vi "transparent IMAQ.vi"() -> ()   [LabVIEW 2015]
uses:
  <vilib>/vision/NI_Vision_Development_Module.lvlib
panel:
  in  "stop":bool
  in  "Transparency":dbl(slide) scale=0.0..100.0
  in  "Background":path=path "C:/Users/Public/Pictures/Sample Pictures/Chrysanthemum.jpg"
  in  "Overlay":path=path "C:/Users/ukrossk/Desktop/QuestionMark.png"
  out "Main Image":T1(plugin-control)
  out "Over Lay":T1(plugin-control)
  out "Image Out":T1(plugin-control)
  # "="
  # "+"
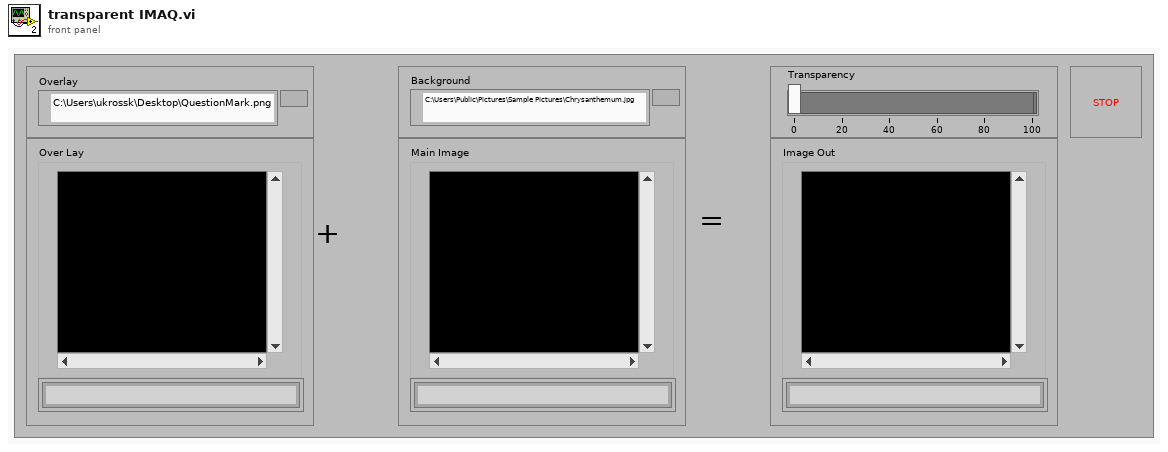
[diagram p1: front panel]
types:
  T1 = typedef "IMAQ Image.ctl" = refnum<image>
  T2 = typedef "Image Type" = u32
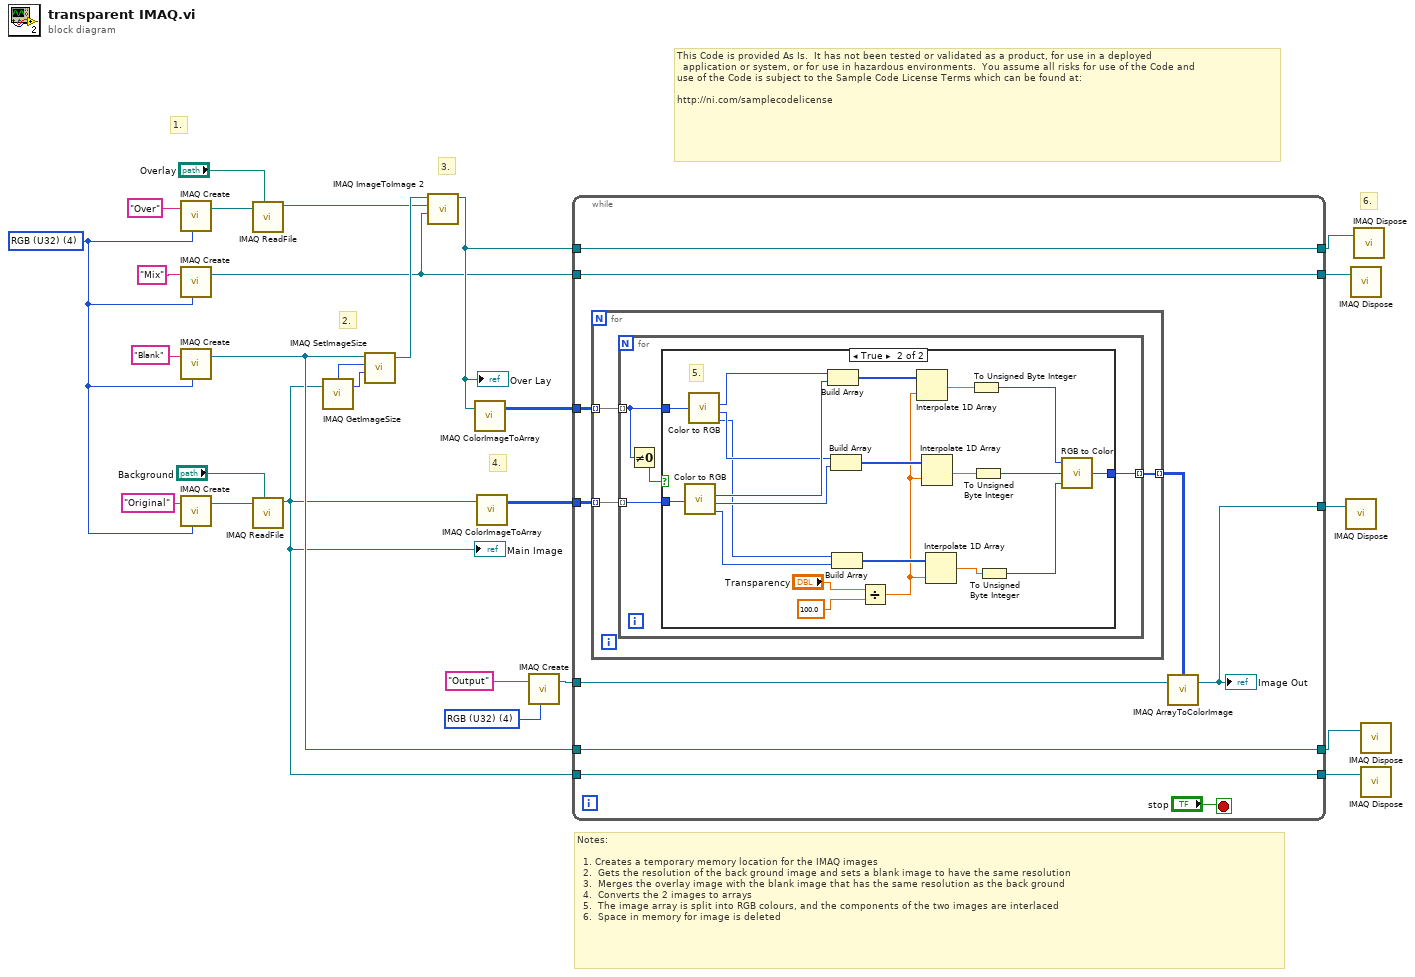
[diagram p0: block diagram]
diagram:
  w11 = T2 4 items=["Grayscale (U8)", "Grayscale (I16)", "Grayscale (SGL)", "Complex (CSG)", "RGB (U32)", "HSL (U32)", "RGB (U64)", "Grayscale (U16)"] ("Image Type")
  w15 = T2 4 items=["Grayscale (U8)", "Grayscale (I16)", "Grayscale (SGL)", "Complex (CSG)", "RGB (U32)", "HSL (U32)", "RGB (U64)", "Grayscale (U16)"] ("Image Type")
  # "6."
  # "4."
  # "3."
  # "2."
  # "1."
  # "Notes:  \n\n  1. Creates a temporary memory location for the IMAQ images\n  2.  Gets the resolution of the back ground image and sets a blank image to have the same resolution\n  3.  Merges the overlay image with the blank image that has the same resolution as the back ground\n  4.  Converts the 2 images to arrays\n  5.  The image array is split into RGB colours, and the components of the two images are interlaced\n  6.  Space in memory for image is deleted"
  # "This Code is provided As Is.  It has not been tested or validated as a product, for use in a deployed\n  application or system, or for use in hazardous environments.  You assume all risks for use of the Code and   \nuse of the Code is subject to the Sample Code License Terms which can be found at: \n\nhttp://ni.com/samplecodelicense"
  n1 = call "IMAQ Create"("Image Name"="Over", "Image Type"=w15) -> ("New Image"=w27:T1)  [unwired: 3 in, 1 out]
  n2 = call "IMAQ Create"("Image Name"="Mix", "Image Type"=w15) -> ("New Image"=w3:T1)  [unwired: 3 in, 1 out]
  n3 = call "IMAQ Create"("Image Name"="Blank", "Image Type"=w15) -> ("New Image"=w9:T1)  [unwired: 3 in, 1 out]
  n4 = call "IMAQ Create"("Image Name"="Original", "Image Type"=w15) -> ("New Image"=w22:T1)  [unwired: 3 in, 1 out]
  n5 = call "IMAQ ReadFile"("File Path"="Overlay", "Image"=w27) -> ("Image Out"=w17:T1)  [unwired: 5 in, 4 out]
  n6 = call "IMAQ ReadFile"("File Path"="Background", "Image"=w22) -> ("Image Out"=w7:T1)  [unwired: 5 in, 4 out]
  "Main Image" <- w7
  n7 = call "IMAQ GetImageSize"("Image"=w7) -> ("Y Resolution"=w20:i32, "X Resolution"=w21:i32)  [unwired: 3 in, 1 out]
  n8 = call "IMAQ SetImageSize"("Y Resolution"=w20, "X Resolution"=w21, "Image"=w9) -> ("Image Out"=w18:T1)  [unwired: 2 in, 1 out]
  n9 = call "IMAQ ImageToImage 2"("Image Dst"=w3, "Image Src (Small)"=w17, "Image Src (Large)"=w18) -> ("Image Dst Out"=w5:T1)  [unwired: 7 in, 1 out]
  "Over Lay" <- w5
  n10 = call "IMAQ ColorImageToArray"("Image"=w5) -> ("Image Pixels (U32)"=w13:u32[][])  [unwired: 3 in, 2 out]
  n11 = call "IMAQ ColorImageToArray"("Image"=w7) -> ("Image Pixels (U32)"=w14:u32[][])  [unwired: 3 in, 2 out]
  n12 = call "IMAQ Create"("Image Name"="Output", "Image Type"=w11) -> ("New Image"=w2:T1)  [unwired: 3 in, 1 out]
  n13 = while {
    tunnel: w14 -> [w37]
    tunnel: w13 -> [w36]
    tunnel: [w34] -> w10
    tunnel: w9 -> [w34]
    tunnel: [w33] -> w8
    tunnel: w7 -> [w33]
    tunnel: [w32] -> w6
    tunnel: w5 -> [w32]
    tunnel: [w31] -> w4
    tunnel: w3 -> [w31]
    tunnel: w2 -> [w29]
    tunnel: [w28] -> w1
    stop <- "stop" stop-if-true
    n14 = for {
      tunnel: w36 -> [w40] mode=indexing
      tunnel: w37 -> [w39] mode=indexing
      tunnel: [w38] -> w30 mode=indexing
      n15 = for {
        tunnel: w40 -> [w42] mode=indexing
        tunnel: w39 -> [w44] mode=indexing
        tunnel: [w43] -> w38 mode=indexing
        n16 = Not Equal To 0?(x=w42) -> (x != 0?=w41:bool)
        n17 = case shown="True" w41 {
          tunnel: w42 -> [_ w66]
          tunnel: w44 -> [w45 w65]
          tunnel: [w45 w49] -> w43
          frame False {
          }
          frame True {
            # "5."
            n18 = call <vilib>:"Color to RGB.vi"("Color"=w65) -> ("R"=w63:u8, "G"=w61:u8, "B"=w59:u8)  [unwired: 1 out]
            n19 = call <vilib>:"Color to RGB.vi"("Color"=w66) -> ("R"=w64:u8, "G"=w62:u8, "B"=w60:u8)  [unwired: 1 out]
            n20 = Build Array(w64, w63) -> (w58:u8[])
            n21 = Build Array(w62, w61) -> (w57:u8[])
            n22 = Build Array(w60, w59) -> (w56:u8[])
            n23 = Divide(x="Transparency", y=100.0) -> (x/y=w48:dbl)
            n24 = Interpolate 1D Array(1:w48, 2:w58) -> (0:w55:dbl)
            n25 = Interpolate 1D Array(1:w48, 2:w57) -> (0:w54:dbl)
            n26 = Interpolate 1D Array(1:w48, 2:w56) -> (0:w53:dbl)
            n27 = To Unsigned Byte Integer(number=w55) -> (unsigned 8bit integer=w52:u8)
            n28 = To Unsigned Byte Integer(number=w54) -> (unsigned 8bit integer=w51:u8)
            n29 = To Unsigned Byte Integer(number=w53) -> (unsigned 8bit integer=w50:u8)
            n30 = call <vilib>:"RGB to Color.vi"("B"=w50, "G"=w51, "R"=w52) -> ("Color"=w49:u32)
          }
        }
      }
    }
    n31 = call "IMAQ ArrayToColorImage"("Image Pixels (U32)"=w30, "Image"=w29) -> ("Image Out"=w28:T1)  [unwired: 3 in, 1 out]
    "Image Out" <- w28
  }
  n32 = call "IMAQ Dispose"("Image"=w1) -> ()  [unwired: 5 in, 1 out]
  n33 = call "IMAQ Dispose"("Image"=w4) -> ()  [unwired: 5 in, 1 out]
  n34 = call "IMAQ Dispose"("Image"=w6) -> ()  [unwired: 5 in, 1 out]
  n35 = call "IMAQ Dispose"("Image"=w10) -> ()  [unwired: 5 in, 1 out]
  n36 = call "IMAQ Dispose"("Image"=w8) -> ()  [unwired: 5 in, 1 out]
